vi "About.vi"(8 "error in (no error)":errorcluster) -> (0 "error IO":errorcluster)   [LabVIEW 2011]
uses:
  <vilib>/Utility/cursorutil.llb/Set Cursor (Icon Pict).vi
  <vilib>/Platform/browser.llb/Open URL in Default Browser (string).vi
panel:
  in  "Link":string="http://decibel.ni.com/content/docs/DOC-18760"
  # "CSV Sequence Player With Point By Point Reporting"
  # "Documentation & Support:"
  # "Version 1.0.0"
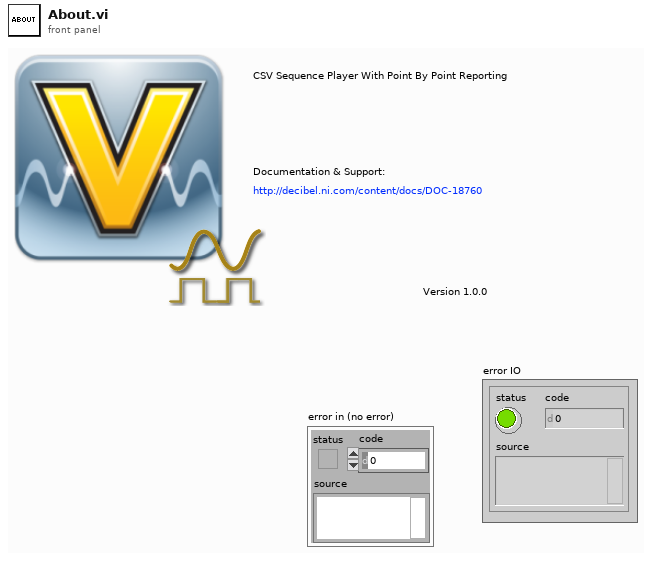
[diagram p1: front panel]
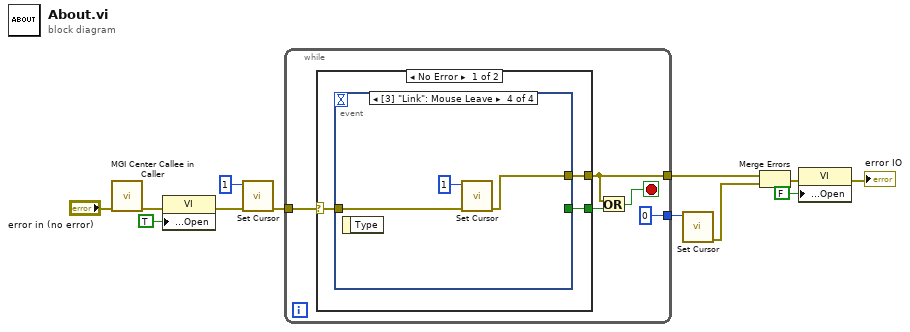
[diagram p0: block diagram]
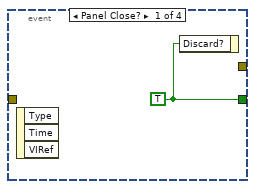
[diagram p2: hidden frame]
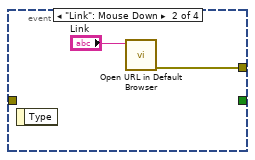
[diagram p3: hidden frame]
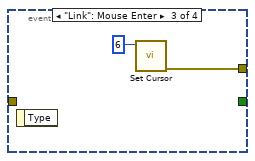
[diagram p4: hidden frame]
diagram:
  n1 = call <userlib>:"MGI Center Callee in Caller.vi"("Error In"="error in (no error)") -> ("Error Out"=w5:errorcluster)  [unwired: 10 in]
  n2 = property on="Property Node" class="VI"(error in=w5, "Front Panel.Open"=TRUE ("Front Panel Window:Open")) -> (error out=w4:errorcluster)  [unwired: 1 in, 1 out]
  n3 = call-poly <vilib>:"Set Cursor.vi"("error in (no error)"=w4, "icon"=u16 1) -> ("error out"=w11:errorcluster)  [unwired: 8 in, 1 out]
  n4 = while {
    tunnel: w11 -> [w15]
    tunnel: [u16 0 ("icon")] -> w10
    tunnel: [w13] -> w9
    stop <- w16 stop-if-true
    n5 = case shown="No Error" w15 {
      selector: w15 -> [w18 w29]
      tunnel: [w20 _] -> w17
      tunnel: [w19 w29] -> w13
      frame No Error {
        n6 = event shown="[3] \"Link\": Mouse Leave" {
          selector: _ -> [_ _ _ _]
          dyn-events: _ -> [_ _ _ _]
          timeout: _ -> [_ _ _ _]
          tunnel: [w21 _ _ _] -> w20
          tunnel: [_ w22 w24 w27] -> w19
          tunnel: w18 -> [_ _ _ w26]
          event Panel Close? {
            w21 = TRUE ("Discard?")
            n7 = event-data() -> ()  [unwired: 1 in, 3 out]
            n8 = event-data("Discard?"=w21) -> ()  [unwired: 1 in, 1 out]
          }
          event "Link": Mouse Down {
            n9 = event-data() -> ()  [unwired: 1 in, 1 out]
            n10 = call-poly <vilib>:"Open URL in Default Browser.vi"("URL"="Link") -> ("error out"=w22:errorcluster)  [unwired: 5 in, 1 out]
          }
          event "Link": Mouse Enter {
            n11 = event-data() -> ()  [unwired: 1 in, 1 out]
            n12 = call-poly <vilib>:"Set Cursor.vi"("icon"=u16 6) -> ("error out"=w24:errorcluster)  [unwired: 9 in, 1 out]
          }
          event "Link": Mouse Leave {
            n13 = event-data() -> ()  [unwired: 1 in, 1 out]
            n14 = call-poly <vilib>:"Set Cursor.vi"("error in (no error)"=w26, "icon"=u16 1) -> ("error out"=w27:errorcluster)  [unwired: 8 in, 1 out]
          }
        }
      }
      frame Error {
      }
    }
    n15 = Or(x=w13, y=w17) -> (x .or. y?=w16:bool)
  }
  n16 = call-poly <vilib>:"Set Cursor.vi"("icon"=w10) -> ("error out"=w8:errorcluster)  [unwired: 9 in, 1 out]
  n17 = Merge Errors(w9, w8) -> (w2:errorcluster)
  n18 = property on="Property Node" class="VI"(error in=w2, "Front Panel.Open"=FALSE ("Front Panel Window:Open")) -> (error out=→"error IO":errorcluster)  [unwired: 1 in, 1 out]
